vi "CODMn参数WR (子VI).vi"(0 "量程选择":enum16{"低量程", "高量程"}(ring), 1 "STEP":enum16{"read", "writekb", "写入消解温度时间"}(ring)=enum."writekb", 2 "方程系数输入":cluster{"X^2":dbl, "X":dbl, "b":dbl} {"X^2" format="%#.4g"; "b" format="%#.4g"; "X" format="%#.4g"}, 3 "消解温度写入":dbl, 4 "恒温时间写入":dbl, 5 "Error in":errorcluster caption="Error in (no error)") -> (14 "方程系数":cluster{"X^2":dbl, "X":dbl, "b":dbl} {"X^2" format="%#.4g"; "b" format="%#.4g"; "X" format="%#.4g"}, 15 "消解温度":dbl, 17 "恒温时间":dbl, 19 "error out":errorcluster)   [LabVIEW 2016]
uses:
  <vilib>/Plasmionique/MB Master/MB_Master_Serial/MB_Master_Serial.lvclass
  C:/Program Files (x86)/National Instruments/LabVIEW 2016/vi.lib/Plasmionique/MB Master/MB_Master/MB_Master.lvclass
  <vilib>/Plasmionique/MB Master/MB Master.lvlib
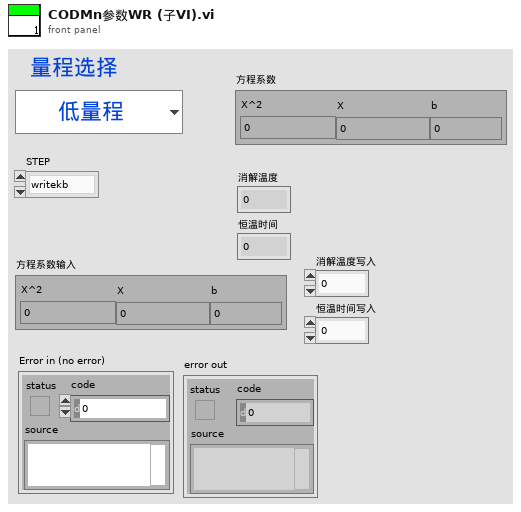
[diagram p1: front panel]
types:
  T1 = cluster{"baud rate (bps)":u32, "stop bits":u16, "parity":u16, "flow control":u16, "timeout":u32, "retries":i32}
  T2 = cluster{"数组 2[0]":sgl, "数组 2[1]":sgl, "数组 2[2]":sgl, "数组 2[3]":sgl, "数组 2[4]":sgl, "数组 2[5]":sgl}
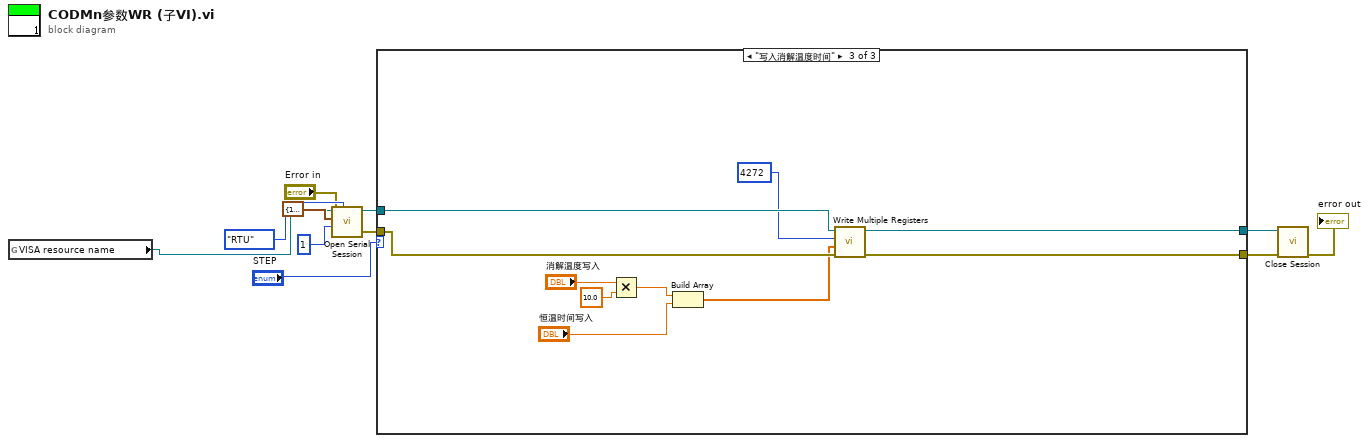
[diagram p0: block diagram]
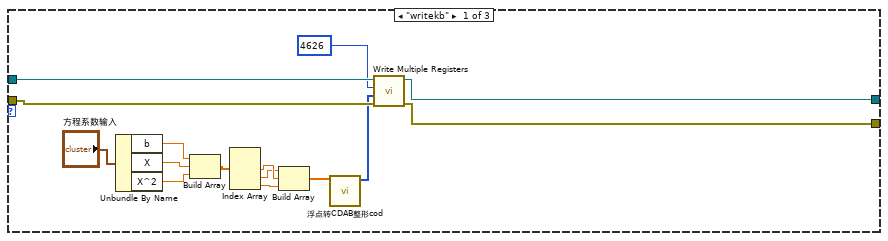
[diagram p2: hidden frame]
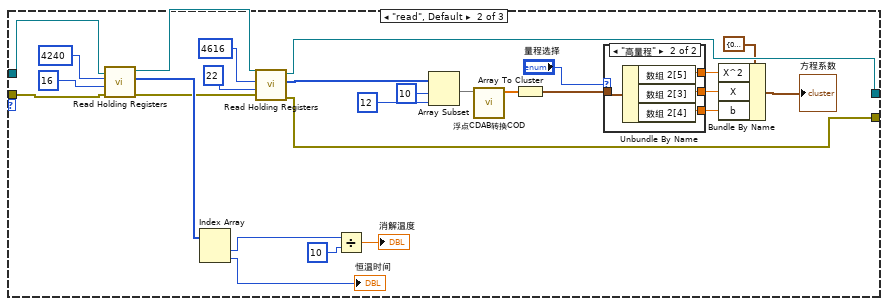
[diagram p3: hidden frame]
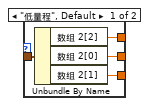
[diagram p4: hidden frame]
diagram:
  n1 = global read "COD浓度全局变量.vi" "VISA resource name"() -> (w8:refnum<visa-resource-name>)
  n2 = call <vilib>:"Open Serial Session.vi"("Mode (RTU)"=enum16{"RTU", "ASCII"}."RTU", "Error in"="Error in", "Slave ID"=u8 1, "Serial Config"=T1 {"baud rate (bps)"=115200, "stop bits"=10, "parity"=0, "flow control"=0, "timeout"=1000, "retries"=1}, "VISA Resource"=w8) -> ("Error out"=w2:errorcluster, "MB_Serial session"=w3:refnum<class "MB_Master_Serial.lvclass">)  [unwired: 5 in]
  n3 = case shown="\"写入消解温度时间\"" "STEP" {
    tunnel: [w13 w53 w65] -> w5
    tunnel: [w12 w52 w64] -> w4
    tunnel: w3 -> [w26 w30 w67]
    tunnel: w2 -> [w25 w29 w66]
    frame "writekb" {
      n4 = Unbundle By Name("方程系数输入") -> ("b"=w20:dbl, "X"=w21:dbl, "X^2"=w22:dbl)
      n5 = Build Array(w20, w21, w22) -> (w23:dbl[])
      n6 = Index Array(array=w23) -> (element #1=w16:dbl, element #2=w15:dbl, element #3=w17:dbl)  [unwired: 3 in]
      n7 = Build Array(w15, w16, w17) -> (w18:dbl[])
      n8 = call "浮点转CDAB整形cod.vi"("浮点数"=w18) -> ("CDAB整形输出"=w14:u16[])  [unwired: 10 in]
      n9 = call <vilib>:"Write Multiple Registers.vi"("error in (no error)"=w25, "values"=w14, "starting address"=u16 4626, "MB session in"=w26) -> ("error out"=w12:errorcluster, "MB session out"=w13:refnum<class "MB_Master_Serial.lvclass">)  [unwired: 6 in]
    }
    frame "read", Default {
      n10 = call <vilib>:"Read Holding Registers.vi"("error in (no error)"=w29, "quantity"=u16 16 ("number of holding registers"), "starting address"=u16 4240, "MB session in"=w30) -> ("error out"=w27:errorcluster, "Registers"=w48:u16[], "MB session out"=w28:refnum<class "MB_Master_Serial.lvclass">)  [unwired: 5 in]
      n11 = Index Array(array=w48) -> (element #1=w49:u16, element #2=→"恒温时间":u16)  [unwired: 2 in]
      n12 = call <vilib>:"Read Holding Registers.vi"("error in (no error)"=w27, "quantity"=u16 22 ("number of holding registers"), "starting address"=u16 4616, "MB session in"=w28) -> ("error out"=w52:errorcluster, "Registers"=w31:u16[], "MB session out"=w53:refnum<class "MB_Master_Serial.lvclass">)  [unwired: 5 in]
      n13 = Divide(x=w49, y=u16 10) -> (x/y=→"消解温度":dbl)
      n14 = Array Subset(array=w31, index=10 ("索引"), length=12 ("长度")) -> (w42:u16[])
      n15 = call "浮点CDAB转换COD.vi"("数组"=w42) -> ("数组 2"=w41:sgl[])  [unwired: 10 in]
      n16 = Array To Cluster(array=w41) -> (cluster=w36:T2)
      n17 = case shown="\"高量程\"" "量程选择" {
        tunnel: w36 -> [w57 w58]
        tunnel: [w56 w61] -> w39
        tunnel: [w55 w60] -> w38
        tunnel: [w54 w59] -> w37
        frame "低量程", Default {
          n18 = Unbundle By Name(w57) -> ("数组 2[2]"=w56:sgl, "数组 2[0]"=w55:sgl, "数组 2[1]"=w54:sgl)
        }
        frame "高量程" {
          n19 = Unbundle By Name(w58) -> ("数组 2[5]"=w61:sgl, "数组 2[3]"=w60:sgl, "数组 2[4]"=w59:sgl)
        }
      }
      n20 = Bundle By Name(cluster=cluster{"X^2":dbl, "X":dbl, "b":dbl} {"X^2"=0.0, "X"=0.0, "b"=0.0} ("方程系数"), "X^2"=w39, "X"=w38, "b"=w37) -> (→"方程系数":cluster{"X^2":dbl, "X":dbl, "b":dbl})
    }
    frame "写入消解温度时间" {
      n21 = Multiply(x="消解温度写入", y=10.0) -> (x*y=w70:dbl)
      n22 = Build Array(w70, "恒温时间写入") -> (w62:dbl[])
      n23 = call <vilib>:"Write Multiple Registers.vi"("error in (no error)"=w66, "values"=w62, "starting address"=u16 4272, "MB session in"=w67) -> ("error out"=w64:errorcluster, "MB session out"=w65:refnum<class "MB_Master_Serial.lvclass">)  [unwired: 6 in]
    }
  }
  n24 = call-dynamic "Close Session.vi"("error in (no error)"=w4, "MB_Serial session"=w5) -> ("error out"=→"error out":errorcluster)  [unwired: 9 in]
